vi "接收数据处理.vi"(6 "接收字符串":string, 9 "reference 3":refnum<vi>, 10 "reference输入":refnum<vi>, 11 "String输入":refnum<vi>) -> ()   [LabVIEW 2016]
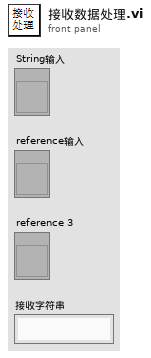
[diagram p1: front panel]
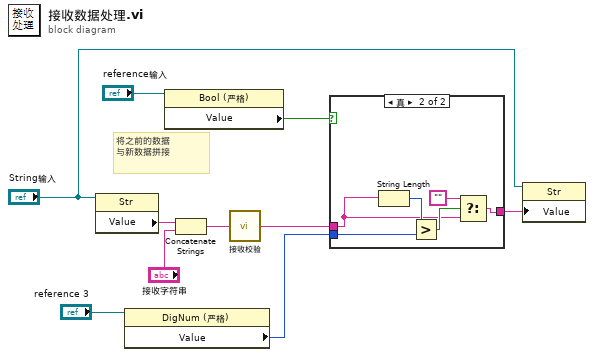
[diagram p0: block diagram]
diagram:
  # "将之前的数据\n与新数据拼接"
  n1 = property class="Str"(reference="String输入") -> ("Value"=w7:string)  [unwired: 1 in, 2 out]
  n2 = property class="DigNum (严格)"(reference="reference 3") -> ("Value"=w9:i32)  [unwired: 1 in, 2 out]
  n3 = property class="Bool (严格)"(reference="reference输入") -> ("Value"=w8:bool)  [unwired: 1 in, 2 out]
  n4 = Concatenate Strings ("连接字符串")(w7, "接收字符串") -> (w6:string)
  n5 = call "接收校验.vi"("字符串"=w6) -> ("s? t:f"=w5:string)
  n6 = case shown="真" w8 {
    tunnel: w5 -> [w11 w15]
    tunnel: [w11 w13] -> w10
    tunnel: w9 -> [_ w12]
    frame False {
    }
    frame True {
      n7 = String Length(string=w15) -> (length=w17:i32)
      n8 = Greater?(x=w17, y=w12) -> (0:w16:bool)
      n9 = Select(t="", s=w16, f=w15) -> (s? t:f=w13:string)
    }
  }
  n10 = property class="Str"(reference="String输入", "Value"=w10) -> ()  [unwired: 1 in, 2 out]
